vi "Current_Filepath.vi"(0 "Filename in":path, 1 "Data Type":string="Calibrations") -> (2 "Filename Out":path, 3 "Directory":path)   [LabVIEW 2011]
uses:
  Globals/Meas_global.vi
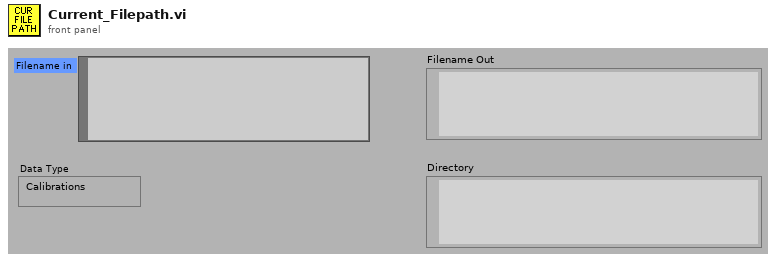
[diagram p1: front panel]
types:
  T1 = typedef "Post_Process.ctl" = enum16{"Take New Data", "Post Process Raw Data File"}
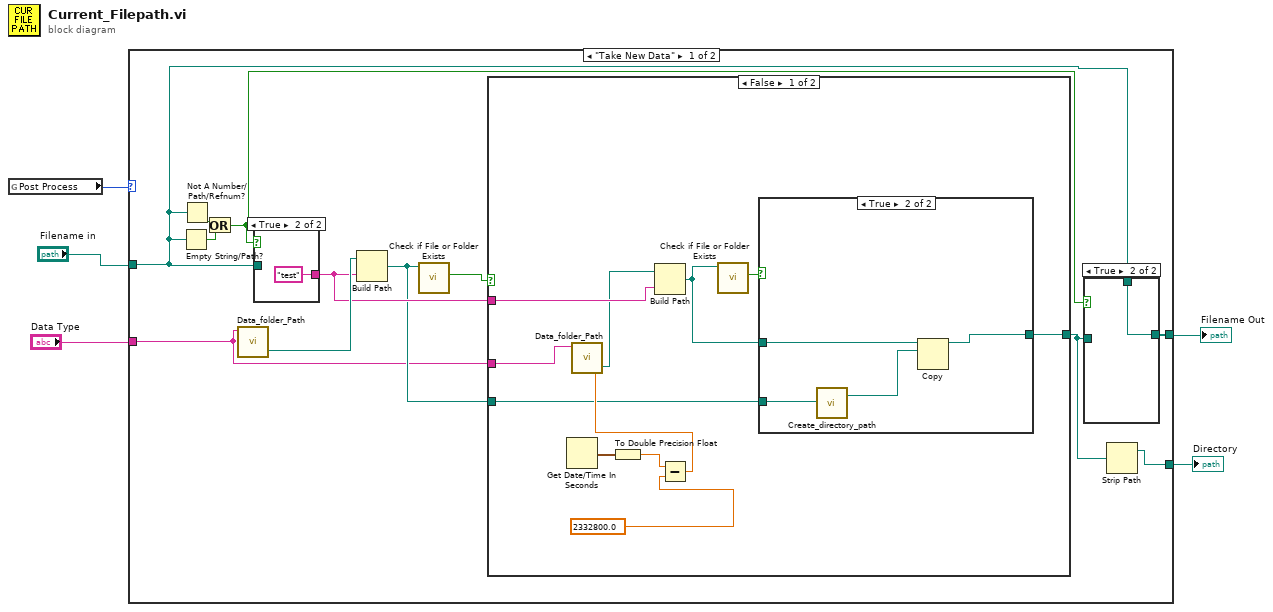
[diagram p0: block diagram]
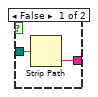
[diagram p3: hidden frame]
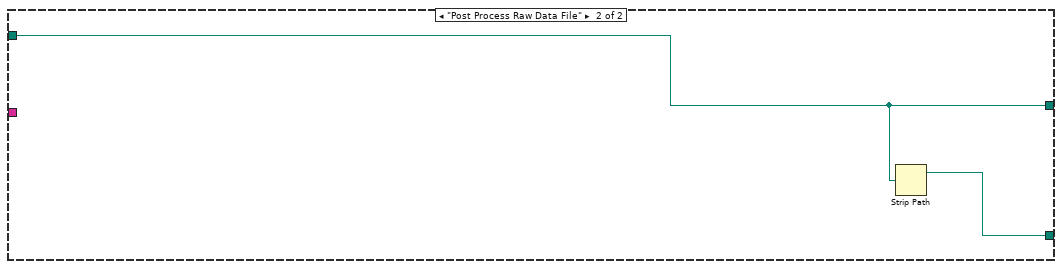
[diagram p6: hidden frame]
diagram:
  n1 = global read "Meas_global.vi" "Post Process"() -> (w2:T1)
  n2 = case shown="\"Take New Data\"" w2 {
    tunnel: "Filename in" -> [w6 w41]
    tunnel: "Data Type" -> [w13 _]
    tunnel: [w9 w41] -> w3
    tunnel: [w7 w40] -> w1
    frame "Take New Data" {
      n3 = Empty String/Path?(string/path=w6) -> (empty?=w11:bool)
      n4 = Not A Number/Path/Refnum?(number/path/refnum=w6) -> (NaN/Path/Refnum?=w12:bool)
      n5 = Or(x=w12, y=w11) -> (x .or. y?=w10:bool)
      n6 = call "Data_folder_Path.vi"("Data Type"=w13) -> ("Data Folder"=w17:path)  [unwired: 4 in]
      n7 = case shown="True" w10 {
        tunnel: [w21 "test" ("name")] -> w15
        tunnel: w6 -> [w20 _]
        frame False {
          n8 = Strip Path(path=w20) -> (name=w21:string)  [unwired: 1 out]
        }
        frame True {
        }
      }
      n9 = Build Path(base path=w17, name or relative path=w15) -> (appended path=w14:path)
      n10 = call <vilib>:"Check if File or Folder Exists.vi"("path"=w14) -> ("file or folder exists?"=w16:bool)  [unwired: 1 in, 9 out]
      n11 = case shown="False" w16 {
        tunnel: w13 -> [w23 _]
        tunnel: w15 -> [w30 _]
        tunnel: w14 -> [w27 w39]
        tunnel: [w25 w39] -> w8
        frame False {
          n12 = Get Date/Time In Seconds() -> (seconds since 1Jan1904=w33:timestamp)
          n13 = To Double Precision Float(number=w33) -> (double precision float=w32:dbl)
          n14 = Subtract(x=w32, y=2332800.0) -> (x-y=w31:dbl)
          n15 = call "Data_folder_Path.vi"("seconds"=w31, "Data Type"=w23) -> ("Data Folder"=w28:path)  [unwired: 3 in]
          n16 = Build Path(base path=w28, name or relative path=w30) -> (appended path=w26:path)
          n17 = call <vilib>:"Check if File or Folder Exists.vi"("path"=w26) -> ("file or folder exists?"=w29:bool)  [unwired: 1 in, 9 out]
          n18 = case shown="True" w29 {
            tunnel: w26 -> [_ w38]
            tunnel: w27 -> [w34 w36]
            tunnel: [w34 w37] -> w25
            frame False {
            }
            frame True {
              n19 = call "Create_directory_path.vi"("Path name"=w36) -> ("Path name Out"=w35:path)  [unwired: 1 in, 1 out]
              n20 = Copy(10:w35, 11:w38) -> (3:w37:path)  [unwired: 3 in, 2 out]
            }
          }
        }
        frame True {
        }
      }
      n21 = case shown="True" w10 {
        tunnel: w8 -> [w18 _]
        tunnel: [w18 w19] -> w9
        tunnel: w6 -> [_ w19]
        frame False {
        }
        frame True {
        }
      }
      n22 = Strip Path(path=w8) -> (stripped path=w7:path)  [unwired: 1 out]
    }
    frame "Post Process Raw Data File" {
      n23 = Strip Path(path=w41) -> (stripped path=w40:path)  [unwired: 1 out]
    }
  }
  "Filename Out" <- w3
  "Directory" <- w1
